vi "Assure Newline at End.vi"(10 "Set End Of Line (F)":bool, 11 "string":string) -> (3 "string out":string)   [LabVIEW 2020, in "infolib.lvlib"]
doc: "Assure a End Of Line is or is not at the end of the string."
uses:
  infolib.lvlib
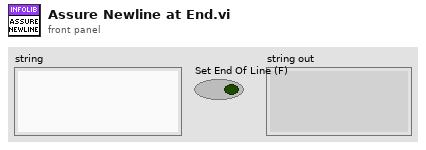
[diagram p1: front panel]
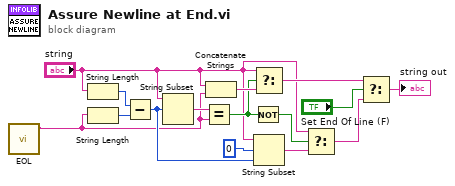
[diagram p0: block diagram]
diagram:
  n1 = call "EOL.vi"() -> ("eol"=w1:string)  [unwired: 11 in]
  n2 = String Length(string="string") -> (length=w14:i32)
  n3 = String Length(string=w1) -> (length=w15:i32)
  n4 = Subtract(x=w14, y=w15) -> (x-y=w5:i32)
  n5 = String Subset(string="string", offset (0)=w5) -> (substring=w2:string)  [unwired: 1 in]
  n6 = Equal?(x=w2, y=w1) -> (x = y?=w9:bool)
  n7 = Concatenate Strings("string", w1) -> (w11:string)
  n8 = Not(x=w9) -> (.not. x?=w10:bool)
  n9 = Select(t="string", s=w9, f=w11) -> (s? t:f=w12:string)
  n10 = String Subset(string="string", offset (0)=0, length (rest)=w5) -> (substring=w3:string)
  n11 = Select(t="string", s=w10, f=w3) -> (s? t:f=w8:string)
  n12 = Select(t=w12, s="Set End Of Line (F)", f=w8) -> (s? t:f=→"string out":string)
